vi "HRTF-Build Matfile Path.vi"(0 "State":T2, 7 "Laterality":T1) -> (4 "path":path, 8 "filestem":string)   [LabVIEW 2015]
uses:
  Typedefs/HRTF-State.ctl
  Typedefs/HRTF-Laterality.ctl
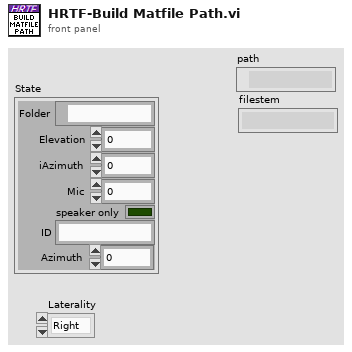
[diagram p1: front panel]
types:
  T1 = typedef "HRTF-Laterality.ctl" = enum16{"Right", "Left"}
  T2 = typedef "HRTF-State.ctl" = cluster{"Folder":path, "Elevation":dbl, "iAzimuth":i32, "Mic":i32, "speaker only":bool, "ID":string, "Azimuth":dbl}
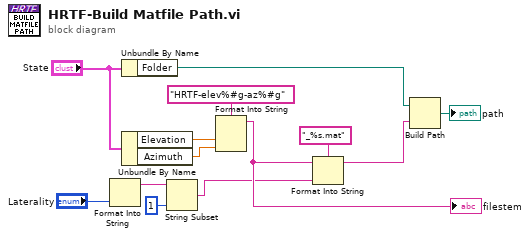
[diagram p0: block diagram]
diagram:
  n1 = Format Into String("Laterality") -> (resulting string=w7:string)  [unwired: 3 in, 1 out]
  n2 = Unbundle By Name("State") -> ("Folder"=w12:path)
  n3 = Unbundle By Name("State") -> ("Elevation"=w10:dbl, "Azimuth"=w11:dbl)
  n4 = String Subset(string=w7, length (rest)=1 ("length (rest)")) -> (substring=w3:string)  [unwired: 1 in]
  n5 = Format Into String(format string="HRTF-elev%#g-az%#g", w10, w11) -> (resulting string=w5:string)  [unwired: 2 in, 1 out]
  "filestem" <- w5
  n6 = Format Into String(format string="_%s.mat", initial string=w5, w3) -> (resulting string=w2:string)  [unwired: 1 in, 1 out]
  n7 = Build Path(base path=w12, name or relative path=w2) -> (appended path=→"path":path)
